vi "Translate.vi"(8 "error in (no error)":errorcluster, 10 "Translation":T1, 11 "Shape in":refnum<class "Shape.lvclass">) -> (0 "error out":errorcluster, 3 "Shape out":refnum<class "Shape.lvclass">)   [LabVIEW 2015, in "LV Image Editor Framework.lvlib" / "Shape.lvclass"]
uses:
  Shape.lvclass
  <vilib>/Utility/miscctls.llb/LVPoint32TypeDef.ctl
  Shape.lvclass/Shape.ctl
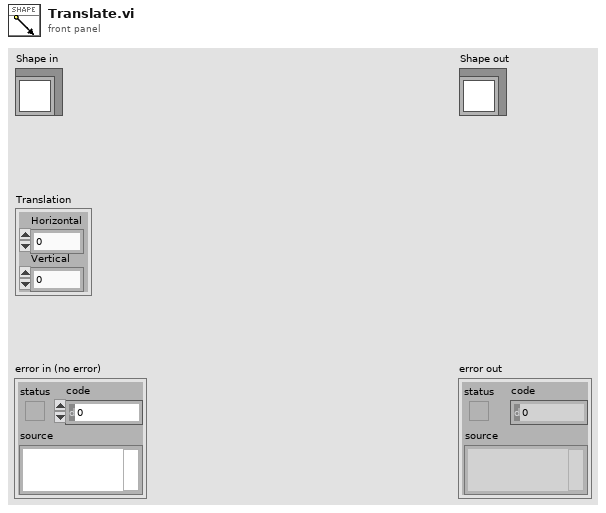
[diagram p1: front panel]
types:
  T1 = typedef "LVPoint32TypeDef.ctl" = cluster{"Horizontal":i32, "Vertical":i32}
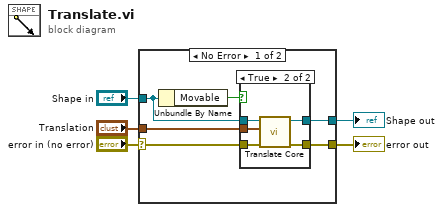
[diagram p0: block diagram]
diagram:
  n1 = case shown="No Error" "error in (no error)" {
    selector: "error in (no error)" -> [w10 w20]
    tunnel: [w9 w20] -> w4
    tunnel: [w11 w19] -> w2
    tunnel: "Shape in" -> [w8 w19]
    tunnel: "Translation" -> [w6 _]
    frame No Error {
      n2 = Unbundle By Name(w8) -> ("Movable"=w7:bool)
      n3 = case shown="True" w7 {
        tunnel: w8 -> [w13 w18]
        tunnel: [w13 w17] -> w11
        tunnel: w10 -> [w12 w16]
        tunnel: [w12 w15] -> w9
        tunnel: w6 -> [_ w14]
        frame False {
        }
        frame True {
          n4 = call-dynamic "Translate Core.vi"("error in (no error)"=w16, "Translation"=w14, "Shape in"=w18) -> ("error out"=w15:errorcluster, "Shape out"=w17:refnum<class "Shape.lvclass">)  [unwired: 7 in]
        }
      }
    }
    frame Error {
    }
  }
  "error out" <- w4
  "Shape out" <- w2
